vi "Fdx Create Session (Tx-Generic).vi"(6 "PortMap":u32, 8 "error in (no error)":errorcluster, 10 "port":u32, 11 "board":u32) -> (0 "error out":errorcluster, 2 "PortInitOut":T1 {"PortConfig" items=["FDX_SINGLE", "FDX_REDUNDANT"]}, 3 "port handle out":u32, 4 "Duplicated":bool, 5 "InstrumentHandle_board out":u32)   [LabVIEW 2020, in "AIM664LV.lvlib"]
doc: "This function creates a session to the board and port and it initializes the port for a Generic Transmit Mode (Tx)."
uses:
  AIM664LV.lvlib
  _controls/hwEntry_actions.ctl
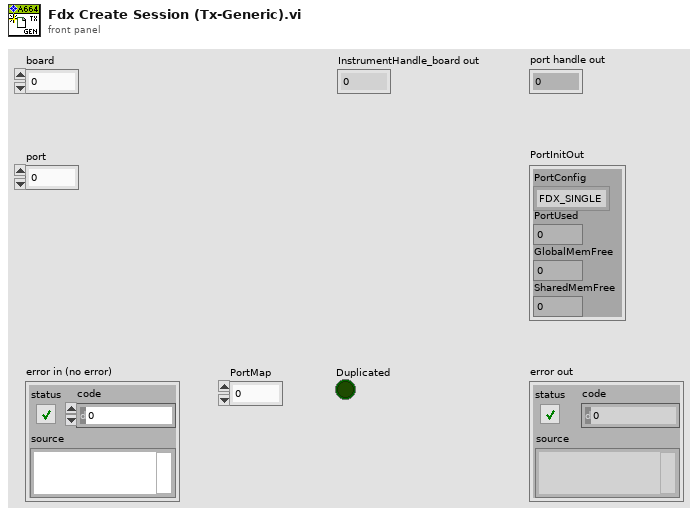
[diagram p1: front panel]
types:
  T1 = cluster{"PortConfig":u32, "PortUsed":u32, "GlobalMemFree":u32, "SharedMemFree":u32}
  T2 = typedef "AIM664LV.lvlib/hwEntry_actions.ctl" = enum16{"Init Port", "Init Board", "Relase Port", "Release Board"}
  T3 = typedef "AIM664LV.lvlib/hwEntry_handleValidityFlag.ctl" = cluster{"boardHandleValid":bool, "portHandleValid":bool}
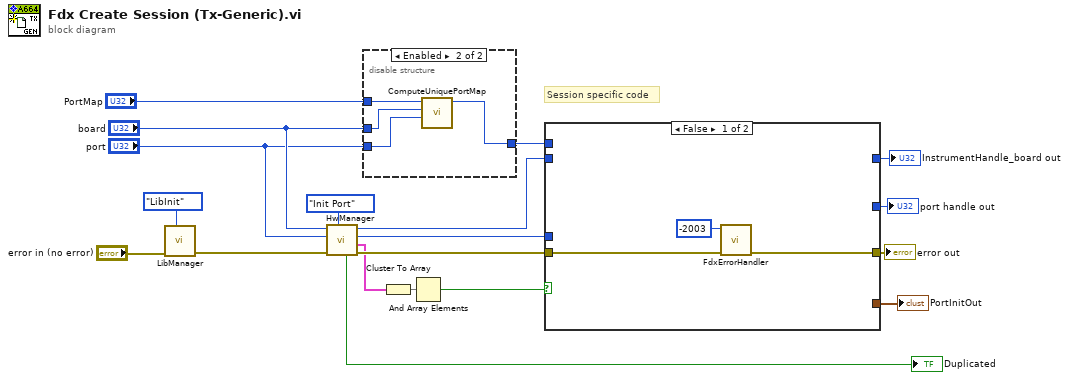
[diagram p0: block diagram]
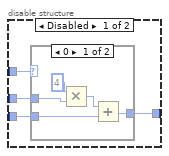
[diagram p2: hidden frame]
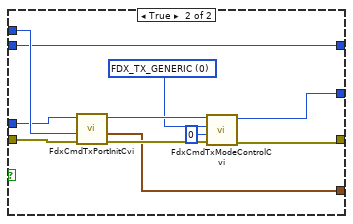
[diagram p4: hidden frame]
diagram:
  # "Session specific code"
  n1 = call "LibManager.vi"("action"=enum16{"LibInit", "LibExit"}."LibInit", "error in (no error)"="error in (no error)") -> ("error out"=w17:errorcluster)  [unwired: 7 in, 2 out]
  n2 = call "HwManager.vi"("action (Init)"=hwEntry_actions."Init Port" ("action"), "error in (no error)"=w17, "port"="port", "board"="board") -> ("error out"=w11:errorcluster, "validityFlag"=w3:T3, "InstrumentHandle_port out"=w9:u32, "InstrumentHandle_board out"=w10:u32, "Duplicated"=→"Duplicated":bool)  [unwired: 3 in]
  n3 = disable-structure shown="Enabled" {
    disable-tunnel: [w23 w30] -> w13
    disable-tunnel: "board" -> [w22 w32]
    disable-tunnel: "port" -> [w21 w31]
    disable-tunnel: "PortMap" -> [w20 w33]
    frame Disabled {
      n4 = case shown="0" w20 {
        selector: w20 -> [_ w29]
        tunnel: [w26 w29] -> w23
        tunnel: w22 -> [w25 _]
        tunnel: w21 -> [w24 _]
        frame 0 {
          n5 = Multiply(x=u32 4, y=w25) -> (x*y=w27:u32)
          n6 = Add(x=w27, y=w24) -> (x+y=w26:u32)
        }
        frame Default {
        }
      }
    }
    frame Enabled {
      n7 = call "ComputeUniquePortMap.vi"("port"=w31, "board"=w32, "PortMap In"=w33) -> ("PortMap out"=w30:u32)  [unwired: 8 in]
    }
  }
  n8 = Cluster To Array(cluster=w3) -> (array=w4:bool[])
  n9 = And Array Elements(Boolean array=w4) -> (logical AND=w2:bool)
  n10 = case shown="False" w2 {
    tunnel: w11 -> [w35 w45]
    tunnel: [w36 w42] -> w16
    tunnel: [_ w43] -> w15
    tunnel: [_ w38] -> w14
    tunnel: w13 -> [_ w40]
    tunnel: w10 -> [_ w37]
    tunnel: w9 -> [_ w39]
    tunnel: [_ w37] -> w5
    frame False {
      n11 = call "FdxErrorHandler.vi"("error in"=w35, "AIM Error"=-2003) -> ("error out"=w36:errorcluster)  [unwired: 9 in]
    }
    frame True {
      w41 = u32 0 items=["FDX_TX_GENERIC", "FDX_TX_REPLAY", "FDX_TX_INDIVIDUAL"] ("TransmitMode")
      n12 = call "FdxCmdTxPortInitCvi.vi"("error in"=w45, "PortMap"=w40, "InstrumentHandle_port"=w39) -> ("error out"=w47:errorcluster, "PortInitOut"=w43:T1, "InstrumentHandle_port"=w44:u32)  [unwired: 6 in]
      n13 = call "FdxCmdTxModeControlCvi.vi"("error in"=w47, "RerosPortDelay"=u32 0, "TransmitMode"=w41, "InstrumentHandle_port"=w44) -> ("error out"=w42:errorcluster, "InstrumentHandle_port"=w38:u32)  [unwired: 6 in]
    }
  }
  "error out" <- w16
  "PortInitOut" <- w15
  "port handle out" <- w14
  "InstrumentHandle_board out" <- w5
